vi "Write subject.vi"(8 "error in (no error)":errorcluster, 10 "Normal Proxy.lvlib:Subject.lvclass":refnum<class "Subject.lvclass">, 11 "OperationLogger (proxy) in":refnum<class "OperationLogger (proxy).lvclass">) -> (0 "error out":errorcluster, 3 "OperationLogger (proxy) out":refnum<class "OperationLogger (proxy).lvclass">)   [LabVIEW 2014, in "Normal Proxy.lvlib" / "OperationLogger (proxy).lvclass"]
uses:
  OperationLogger (proxy).lvclass
  Subject/Subject.lvclass
  OperationLogger (proxy).lvclass/OperationLogger (proxy).ctl
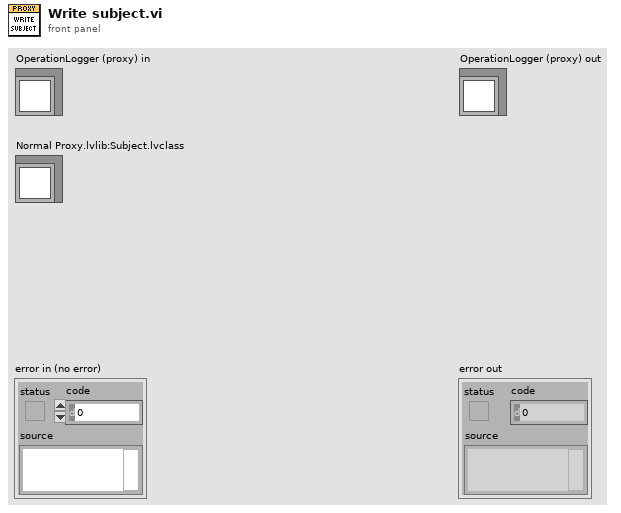
[diagram p1: front panel]
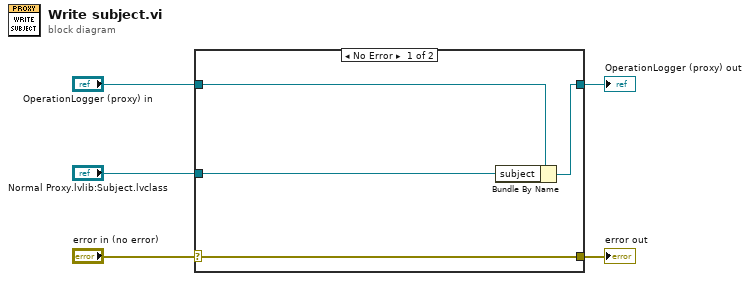
[diagram p0: block diagram]
diagram:
  n1 = case shown="No Error" "error in (no error)" {
    selector: "error in (no error)" -> [w9 w10]
    tunnel: [w9 w10] -> w4
    tunnel: [w7 w11] -> w2
    tunnel: "OperationLogger (proxy) in" -> [w8 w11]
    tunnel: "Normal Proxy.lvlib:Subject.lvclass" -> [w6 _]
    frame No Error {
      n2 = Bundle By Name(cluster=w8, "subject"=w6) -> (w7:refnum<class "OperationLogger (proxy).lvclass">)
    }
    frame Error {
    }
  }
  "error out" <- w4
  "OperationLogger (proxy) out" <- w2
